vi "funny average complex.vi"(10 "in":cdb[](array[numeric])) -> (2 "Out":cdb[](array[numeric]))   [LabVIEW 2020]
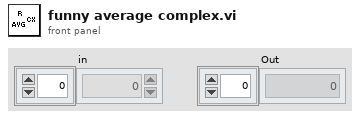
[diagram p1: front panel]
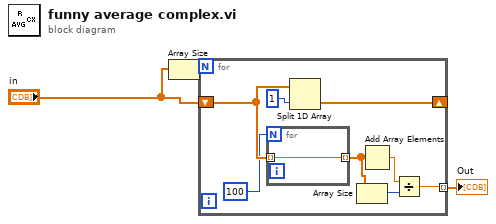
[diagram p0: block diagram]
diagram:
  n1 = Array Size(array="in") -> (size(s)=w3:i32)
  n2 = for {
    N: w3 -> [_]
    shift-right: [w9] -> _
    shift-left: "in" -> [w11]
    tunnel: [w6] -> w1 mode=indexing
    n3 = for {
      N: 100 -> [_]
      tunnel: w11 -> [w12] mode=indexing
      tunnel: [w12] -> w5 mode=indexing
    }
    n4 = Split 1D Array(array=w11, index=1) -> (second subarray=w9:cdb[])  [unwired: 1 out]
    n5 = Array Size(array=w5) -> (size(s)=w4:i32)
    n6 = Add Array Elements(numeric array=w5) -> (sum=w8:cdb)
    n7 = Divide(x=w8, y=w4) -> (x/y=w6:cdb)
  }
  "Out" <- w1
